vi "CT-Test (sweep).vi"() -> ()   [LabVIEW 2015]
uses:
  Utility VIs/Math VIs/FFT x(t) to dB,Degrees (1D).vi
  HCT-Phase Enum.ctl
  HCT-Params.ctl
panel:
  out "Elapsed time (ms)":u32
  in  "F0 (Hz)":dbl[](array[numeric])
  out "Time":cluster{"Array":dbl[], "Array":dbl[]}[](graph)
  out "Freq":cluster{"Array":dbl[], "Array":dbl[]}(graph)
  in  "Frame size (ms)":dbl=100.0
  in  "Fs (Hz)":dbl=50000.0
  in  "HCT Params":T1={"F0 (Hz)"=500.0, "Band"={"Flow (Hz)"=800.0, "Fhigh (Hz)"=8000.0}, "Phase"=enum."Cosine", "Min F0 (Hz)"=0.0, "Max F0 (Hz)"=0.0}
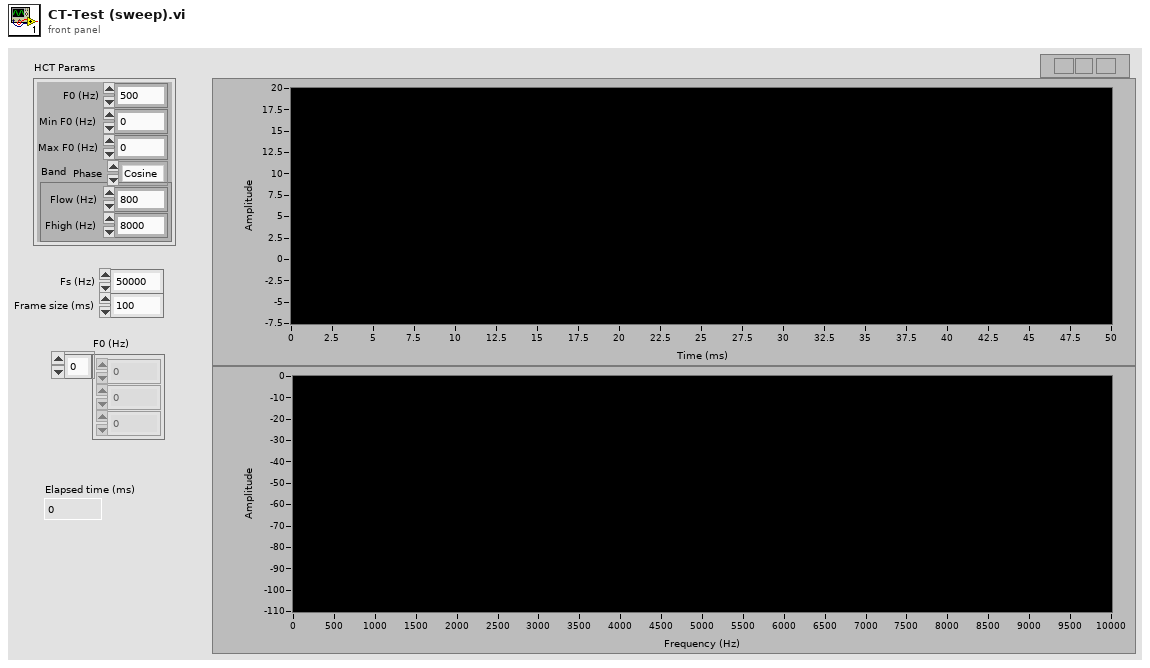
[diagram p1: front panel]
types:
  T1 = typedef "HCT-Params.ctl" = cluster{"F0 (Hz)":dbl, "Band":cluster{"Flow (Hz)":dbl, "Fhigh (Hz)":dbl}, "Phase":T2, "Min F0 (Hz)":dbl, "Max F0 (Hz)":dbl}
  T2 = typedef "HCT-Phase Enum.ctl" = enum16{"Cosine", "Random", "Alternating"}
  T3 = typedef "HCT-Runtime Data.ctl" = cluster{"Ncomp":i32, "MinHarm":i32, "Phase":dbl[], "Amplitude":dbl[], "Npts/frame":i32, "Last F0":dbl, "Fmin":dbl, "Fmax":dbl}
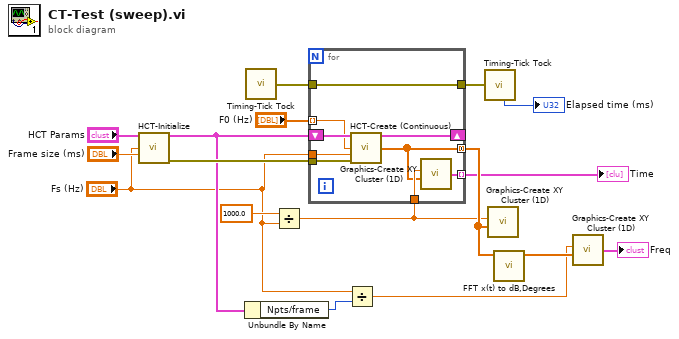
[diagram p0: block diagram]
diagram:
  n1 = call "HCT-Initialize.vi"("HCT Params"="HCT Params", "Fs (Hz)"="Fs (Hz)", "Frame size (ms)"="Frame size (ms)") -> ("HCT Runtime"=w6:T3, "error out"=w15:errorcluster)  [unwired: 11 in]
  n2 = Unbundle By Name(w6) -> ("Npts/frame"=w12:i32)
  n3 = call "Timing-Tick Tock.vi"() -> ("error out"=w3:errorcluster)  [unwired: 6 in, 1 out]
  n4 = Divide(x=1000.0, y="Fs (Hz)") -> (x/y=w4:dbl)
  n5 = for {
    tunnel: w15 -> [w26]
    tunnel: [w20] -> w13 mode=concatenating
    tunnel: "Fs (Hz)" -> [w25]
    tunnel: "F0 (Hz)" -> [w23] mode=indexing
    shift-right: [w22] -> _
    shift-left: w6 -> [w24]
    tunnel: w4 -> [w21]
    tunnel: [w19] -> w7 mode=indexing
    tunnel: [w18] -> w2
    tunnel: w3 -> [w18]
    n6 = call "HCT-Create (Continuous).vi"("HCT Runtime in"=w24, "F0 (Hz)"=w23, "Fs (Hz)"=w25, "error in (no error)"=w26) -> ("HCT Runtime out"=w22:T3, "HCT"=w20:dbl[])  [unwired: 9 in, 1 out]
    n7 = call "Graphics-Create XY Cluster (1D).vi"("Array"=w20, "dx"=w21) -> ("XY cluster"=w19:cluster{"Array":dbl[], "Array":dbl[]})  [unwired: 2 in]
  }
  "Time" <- w7
  n8 = Divide(x="Fs (Hz)", y=w12) -> (x/y=w10:dbl)
  n9 = call "Timing-Tick Tock.vi"("error in (no error)"=w2) -> ("Elapsed time (ms)"=→"Elapsed time (ms)":u32)  [unwired: 5 in, 1 out]
  n10 = call "Graphics-Create XY Cluster (1D).vi"("Array"=w13, "dx"=w4) -> ()  [unwired: 2 in, 1 out]
  n11 = call-poly "FFT x(t) to dB,Degrees.vi"("X"=w13) -> ("+Freq. Mag of FFT (dB rms)"=w11:dbl[])  [unwired: 8 in, 2 out]
  n12 = call "Graphics-Create XY Cluster (1D).vi"("Array"=w11, "dx"=w10) -> ("XY cluster"=→"Freq":cluster{"Array":dbl[], "Array":dbl[]})  [unwired: 2 in]
